vi "saveGraph.vi"(0 "reference":refnum<class "Graph.lvclass">, 1 "filePath":path, 2 "diagramType":T2, 5 "error in (no error)":errorcluster, 6 "ExportType(Normal)":T1) -> (14 "reference out":refnum<class "Graph.lvclass">, 15 "succeeded":bool, 19 "error out":errorcluster)   [LabVIEW 2014, in "Graph.lvclass"]
doc: "Save to File"
uses:
  <resource>/Framework/Providers/Open_GDS/UML/Graph_class/Graph.lvclass
  <resource>/Framework/Providers/Open_GDS/UML/Graph_class/private/diagramType.ctl
  <resource>/Framework/Providers/Open_GDS/UML/Graph_class/SaveTypes.ctl
  <resource>/Framework/Providers/Open_GDS/UML/Graph_class/private/FileSaveVersionType.ctl
  <resource>/Framework/Providers/Open_GDS/UML/AbstractNode_class/AbstractNode.lvclass
  <resource>/Framework/Providers/Open_GDS/UML/AbstractEdge_class/AbstractEdge.lvclass
panel:
  in  "Old":bool
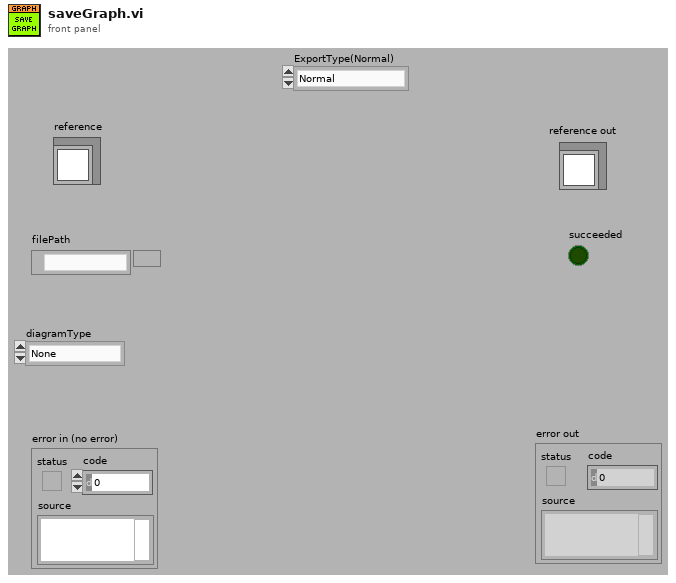
[diagram p1: front panel]
types:
  T1 = typedef "Graph.lvclass/SaveTypes.ctl" = enum16{"Normal", "XMI"}
  T2 = typedef "Graph.lvclass/diagramType.ctl" = enum16{"None", "Class", "Sequency", "State", "UseCase", "DQMH-Module"}
  T3 = cluster{"nodeInfo":cluster{"NodeType":string[], "ParentIndex":i32[], "ChildernIndexies":cluster{i32[]}[], "FlattenData":string[]}, "edgeInfo":cluster{"EdgeType":string[], "StartNodeIndex":i32[], "EndNodeIndex":i32[], "FlattenData":string[]}, "Succeeded":bool, "DiagramData":string}
  T4 = typedef "Graph.lvclass/ObjectAttributes.ctl" = cluster{"nodes":refnum<class "AbstractNode.lvclass">[], "edges":refnum<class "AbstractEdge.lvclass">[], "nodesToBeRemoved":refnum<class "AbstractNode.lvclass">[], "edgesToBeRemoved":refnum<class "AbstractEdge.lvclass">[], "needsLayout":bool, "LayoutNodes":refnum<class "AbstractNode.lvclass">[]}
  T5 = cluster{"children":refnum<class "AbstractNode.lvclass">[]}
  T6 = cluster{"NodeType":string[], "ParentIndex":i32[], "ChildernIndexies":cluster{i32[]}[], "FlattenData":string[]}
  T7 = cluster{"EdgeType":string[], "StartNodeIndex":i32[], "EndNodeIndex":i32[], "FlattenData":string[]}
  T8 = typedef "Graph.lvclass/FileSaveVersionType.ctl" = enum16{"A", "B"}
  T9 = cluster{"TYPEDEF-FileSaveVersion":T8, "diagramType":T2, "DiagramData":string, "nodeInfo":cluster{"NodeType":string[], "ParentIndex":i32[], "ChildernIndexies":cluster{i32[]}[], "FlattenData":string[]}, "edgeInfo":cluster{"EdgeType":string[], "StartNodeIndex":i32[], "EndNodeIndex":i32[], "FlattenData":string[]}}
  T10 = cluster{"diagramType":T2, "nodeInfo":cluster{"NodeType":string[], "ParentIndex":i32[], "ChildernIndexies":cluster{i32[]}[], "FlattenData":string[]}, "edgeInfo":cluster{"EdgeType":string[], "StartNodeIndex":i32[], "EndNodeIndex":i32[], "FlattenData":string[]}}
  T11 = enum16{"open", "replace", "create", "open or create", "replace or create", "replace or create with confirmation"}
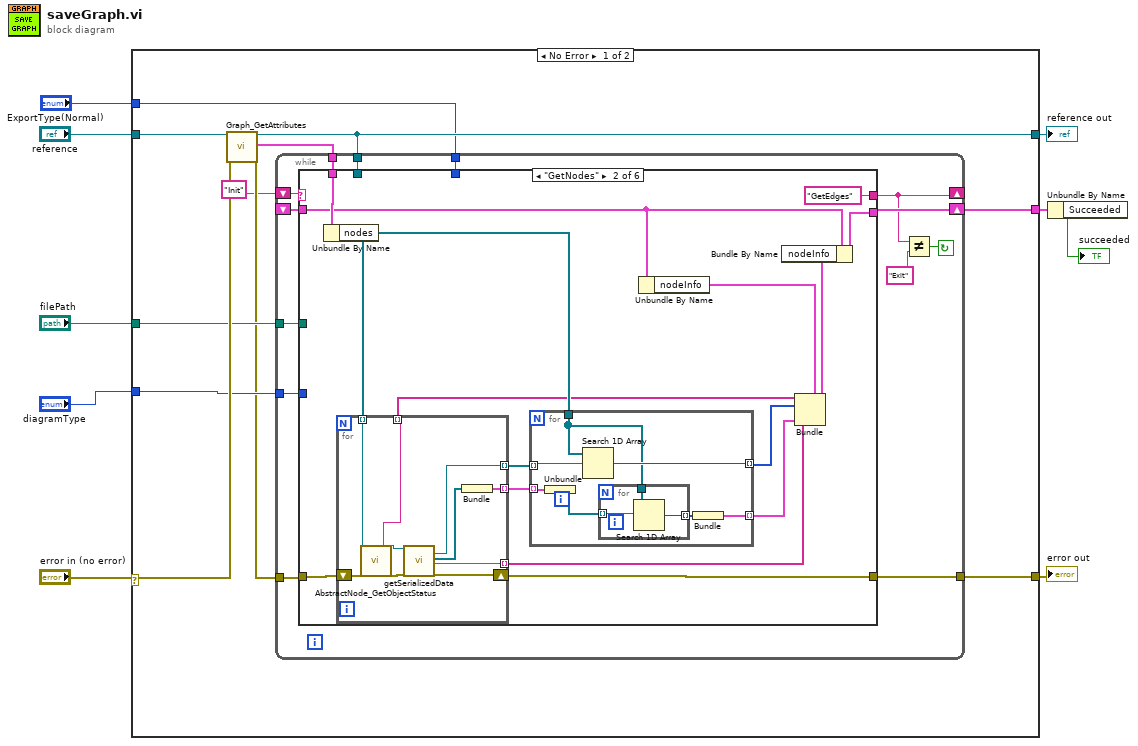
[diagram p0: block diagram]
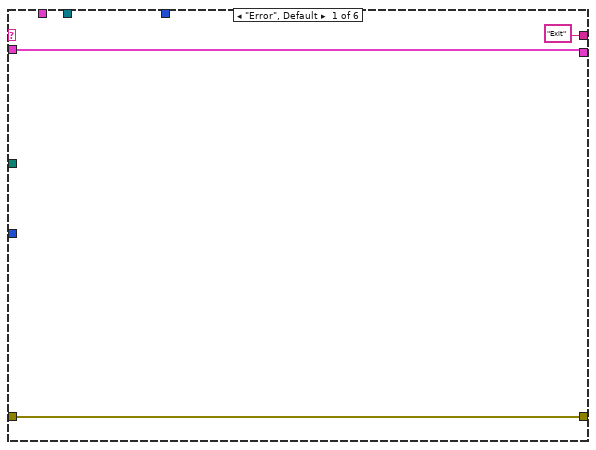
[diagram p2: hidden frame]
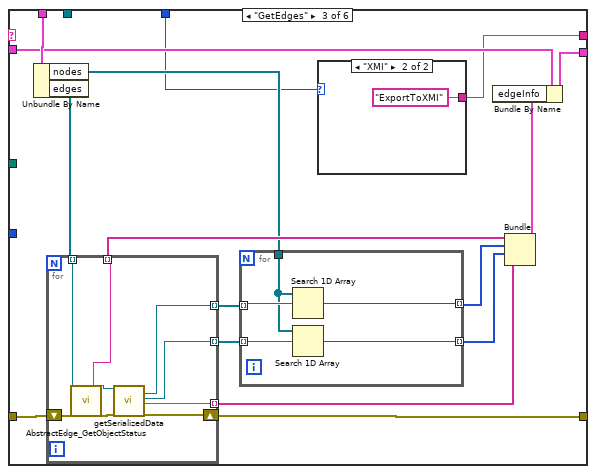
[diagram p3: hidden frame]
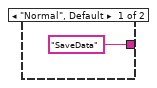
[diagram p4: hidden frame]
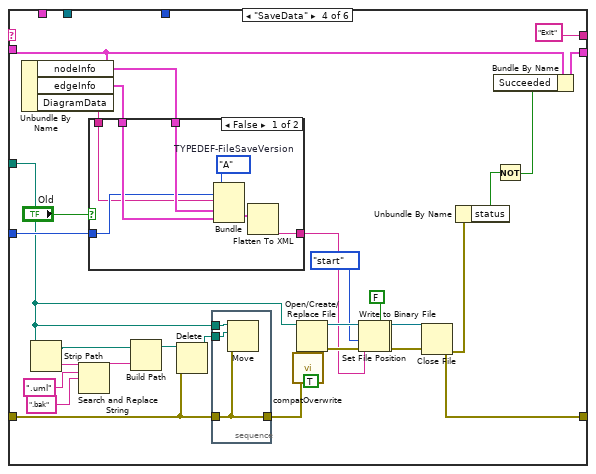
[diagram p5: hidden frame]
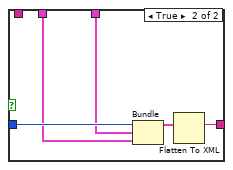
[diagram p6: hidden frame]
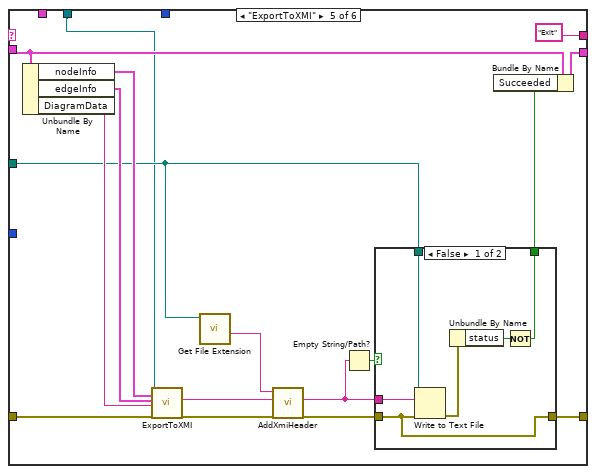
[diagram p7: hidden frame]
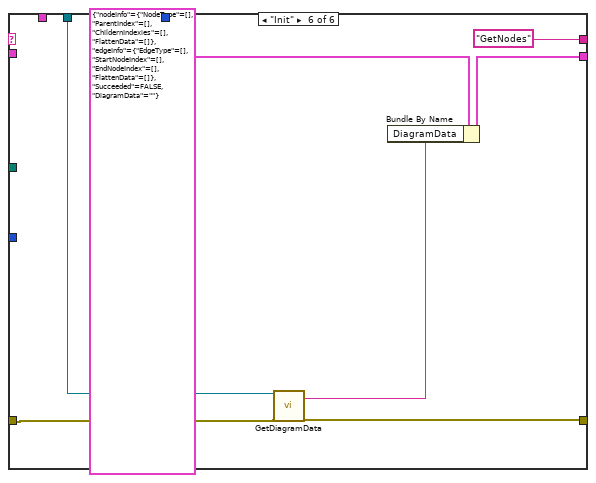
[diagram p9: hidden frame]
diagram:
  n1 = case shown="No Error" "error in (no error)" {
    selector: "error in (no error)" -> [w17 w180]
    tunnel: "reference" -> [w20 w181]
    tunnel: [w19 w180] -> w8
    tunnel: [w18 w181] -> w7
    tunnel: "filePath" -> [w16 _]
    tunnel: "diagramType" -> [w15 _]
    tunnel: [w14 _] -> w3
    tunnel: "ExportType(Normal)" -> [w13 _]
    frame No Error {
      n2 = call <resource>:"Graph_GetAttributes.vi"("reference in"=w20, "error in (no error)"=w17) -> ("reference out"=w18:refnum<class "Graph.lvclass">, "Data"=w10:T4, "error out"=w12:errorcluster)  [unwired: 1 in, 14 out]
      n3 = while {
        tunnel: w10 -> [w33]
        tunnel: w12 -> [w32]
        tunnel: w15 -> [w31]
        tunnel: w16 -> [w30]
        tunnel: [w29] -> w19
        shift-right: [w24] -> _
        shift-left: "Init" -> [w28]
        shift-right: [w27] -> w14
        shift-left: _ -> [w23]
        tunnel: w18 -> [w22]
        tunnel: w13 -> [w21]
        stop <- w25 continue-if-true
        n4 = case shown="\"GetNodes\"" w28 {
          tunnel: w33 -> [_ w51 w86 _ _ _]
          tunnel: w32 -> [w36 w50 w85 w111 w162 w176]
          tunnel: w31 -> [_ _ _ w132 _ _]
          tunnel: w30 -> [_ _ _ w109 w151 _]
          tunnel: [w36 w44 w81 w125 w157 w175] -> w29
          tunnel: [w34 w40 w77 w121 w164 w177] -> w27
          tunnel: ["Exit" ("y") "GetEdges" w71 "Exit" ("y") "Exit" ("y") "GetNodes"] -> w24
          tunnel: w23 -> [w34 w38 w79 w120 w163 _]
          tunnel: w22 -> [_ _ _ _ w149 w173]
          tunnel: w21 -> [_ _ w72 _ _ _]
          frame "Error", Default {
          }
          frame "GetNodes" {
            n5 = Unbundle By Name(w51) -> ("nodes"=w43:refnum<class "AbstractNode.lvclass">[])
            n6 = for {
              shift-right: [w63] -> w44
              shift-left: w50 -> [w70]
              tunnel: w43 -> [w66] mode=indexing
              tunnel: [w69] -> w49 mode=indexing
              tunnel: [w67] -> w48 mode=indexing
              tunnel: [w64] -> w45 mode=indexing
              tunnel: [w62] -> w42 mode=indexing
              n7 = call <resource>:"AbstractNode_GetObjectStatus.vi"("reference in"=w66) -> ("Class name"=w62:string, "reference out"=w65:refnum<class "AbstractNode.lvclass">)  [unwired: 1 in, 16 out]
              n8 = call-dynamic "getSerializedData.vi"("reference"=w65, "error in (no error)"=w70) -> ("parent"=w69:refnum<class "AbstractNode.lvclass">, "children"=w68:refnum<class "AbstractNode.lvclass">[], "xmlOut"=w64:string, "error out"=w63:errorcluster)  [unwired: 13 in, 1 out]
              n9 = Bundle("children"=w68) -> (w67:T5)  [unwired: 1 in]
            }
            n10 = for {
              tunnel: w49 -> [w57] mode=indexing
              tunnel: w48 -> [w58] mode=indexing
              tunnel: [w56] -> w47 mode=indexing
              tunnel: [w53] -> w46 mode=indexing
              tunnel: w43 -> [w52]
              n11 = Unbundle(w58) -> ("children"=w55:refnum<class "AbstractNode.lvclass">[])
              n12 = Search 1D Array(1D array=w52, element=w57) -> (index of element=w56:i32)  [unwired: 1 out]
              n13 = for {
                tunnel: w55 -> [w60] mode=indexing
                tunnel: w52 -> [w61]
                tunnel: [w59] -> w54 mode=indexing
                n14 = Search 1D Array(1D array=w61, element=w60) -> (index of element=w59:i32)  [unwired: 1 out]
              }
              n15 = Bundle(w54) -> (w53:cluster{i32[]})  [unwired: 1 in]
            }
            n16 = Unbundle By Name(w38) -> ("nodeInfo"=w37:T6)
            n17 = Bundle(cluster=w37, "NodeType"=w42, "ParentIndex"=w47, "ChildernIndexies"=w46, "FlattenData"=w45) -> (w41:T6)
            n18 = Bundle By Name(cluster=w38, "nodeInfo"=w41) -> (w40:T3)
          }
          frame "GetEdges" {
            n19 = Unbundle By Name(w86) -> ("nodes"=w76:refnum<class "AbstractNode.lvclass">[], "edges"=w75:refnum<class "AbstractEdge.lvclass">[])
            n20 = for {
              shift-right: [w95] -> w81
              shift-left: w85 -> [w101]
              tunnel: w75 -> [w99] mode=indexing
              tunnel: [w100] -> w84 mode=indexing
              tunnel: [w96] -> w82 mode=indexing
              tunnel: [w94] -> w80 mode=indexing
              tunnel: [w97] -> w74 mode=indexing
              n21 = call <resource>:"AbstractEdge_GetObjectStatus.vi"("reference in"=w99) -> ("Class name"=w94:string, "reference out"=w98:refnum<class "AbstractEdge.lvclass">)  [unwired: 1 in, 16 out]
              n22 = call-dynamic "getSerializedData.vi"("reference"=w98, "error in (no error)"=w101) -> ("startNode"=w100:refnum<class "AbstractNode.lvclass">, "endNode"=w97:refnum<class "AbstractNode.lvclass">, "xmlOut"=w96:string, "error out"=w95:errorcluster)  [unwired: 13 in, 1 out]
            }
            n23 = for {
              tunnel: w84 -> [w93] mode=indexing
              tunnel: [w92] -> w83 mode=indexing
              tunnel: w76 -> [w91]
              tunnel: w74 -> [w90] mode=indexing
              tunnel: [w89] -> w73 mode=indexing
              n24 = Search 1D Array(1D array=w91, element=w93) -> (index of element=w92:i32)  [unwired: 1 out]
              n25 = Search 1D Array(1D array=w91, element=w90) -> (index of element=w89:i32)  [unwired: 1 out]
            }
            n26 = case shown="\"XMI\"" w72 {
              tunnel: ["SaveData" "ExportToXMI"] -> w71
              frame "Normal", Default {
              }
              frame "XMI" {
              }
            }
            n27 = Bundle(w80, w83, w73, w82) -> (w78:cluster{string[], i32[], i32[], string[]})  [unwired: 1 out]
            n28 = Bundle By Name(cluster=w79, "edgeInfo"=w78) -> (w77:T3)
          }
          frame "SaveData" {
            n29 = Unbundle By Name(w120) -> ("nodeInfo"=w131:T6, "edgeInfo"=w130:T7, "DiagramData"=w107:string)
            n30 = Strip Path(path=w109) -> (stripped path=w118:path, name=w117:string)
            n31 = Search and Replace String(input string=w117, search string=".uml", replace string=".bak" ("replace string (\"\")")) -> (result string=w114:string)  [unwired: 1 in, 7 out]
            n32 = case shown="False" "Old" {
              tunnel: w132 -> [w137 w145]
              tunnel: w131 -> [w139 w144]
              tunnel: w130 -> [w138 w143]
              tunnel: w107 -> [w134 _]
              tunnel: [w135 w141] -> w106
              frame False {
                w140 = FileSaveVersionType."A"  # TYPEDEF-FileSaveVersion
                n33 = Bundle("TYPEDEF-FileSaveVersion"=w140, "diagramType"=w137, "DiagramData"=w134, "nodeInfo"=w139, "edgeInfo"=w138) -> (w136:T9)  [unwired: 1 out]
                n34 = Flatten To XML(anything=w136) -> (xml string=w135:string)
              }
              frame True {
                n35 = Bundle("diagramType"=w145, "nodeInfo"=w144, "edgeInfo"=w143) -> (w142:T10)  [unwired: 1 out]
                n36 = Flatten To XML(anything=w142) -> (xml string=w141:string)
              }
            }
            n37 = Build Path(base path=w118, name or relative path=w114) -> (appended path=w113:path)
            n38 = Delete(path (use dialog)=w113, error in=w111) -> (deleted path=w112:path)  [unwired: 5 out]
            n39 = stacked-sequence {
              tunnel: w109 -> [w148]
              tunnel: w112 -> [w147]
              tunnel: w111 -> [w146]
              tunnel: [w146] -> w110
              frame #0 {
                n40 = Move(source path=w148, error in=w146, 10:w147) -> ()  [unwired: 5 out]
              }
            }
            n41 = call <vilib>:"compatOverwrite.vi"("overwrite (F)"=TRUE) -> ("overwrite?"=w105:T11)
            n42 = Open/Create/Replace File(file path (use dialog)=w109, error in=w110, operation (0:open)=w105) -> (refnum out=w128:refnum<file>, error out=w129:errorcluster)  [unwired: 3 in, 1 out]
            n43 = Set File Position(refnum=w128, from (0:start)=enum16{"start", "end", "current"}."start" ("pos mode (0:2)"), error in=w129) -> (refnum out=w104:refnum<file>, error out=w103:errorcluster)  [unwired: 1 out]
            n44 = Write to Binary File(file (use dialog)=w104, data=w106, error in=w103, 5:FALSE ("prepend array or string size? (T)")) -> (refnum out=w126:refnum<file>, error out=w127:errorcluster)  [unwired: 3 out]
            n45 = Close File(refnum=w126, error in=w127) -> (error out=w125:errorcluster)  [unwired: 1 out]
            n46 = Unbundle By Name(w125) -> ("status"=w122:bool)
            n47 = Not(x=w122) -> (.not. x?=w119:bool)
            n48 = Bundle By Name(cluster=w120, "Succeeded"=w119) -> (w121:T3)
          }
          frame "ExportToXMI" {
            n49 = Unbundle By Name(w163) -> ("nodeInfo"=w161:T6, "edgeInfo"=w160:T7, "DiagramData"=w159:string)
            n50 = call-dynamic "ExportToXMI.vi"("reference"=w149, "nodeInfo"=w161, "edgeInfo"=w160, "DiagramData"=w159, "error in (no error)"=w162) -> ("XMIText"=w155:string, "error out"=w154:errorcluster)  [unwired: 12 in, 1 out]
            n51 = call <vilib>:"Get File Extension.vi"("file"=w151) -> ("filename without extension"=w150:string)  [unwired: 1 in, 9 out]
            n52 = call <resource>:"AddXmiHeader.vi"("error in (no error)"=w154, "XmiContent"=w155, "DiagramName"=w150) -> ("error out"=w153:errorcluster, "XmiDocument"=w152:string)  [unwired: 7 out]
            n53 = Empty String/Path?(string/path=w152) -> (empty?=w158:bool)
            n54 = case shown="False" w158 {
              tunnel: w153 -> [w169 w172]
              tunnel: [w169 w172] -> w157
              tunnel: [w166 _] -> w156
              tunnel: w151 -> [w171 _]
              tunnel: w152 -> [w170 _]
              frame False {
                n55 = Write to Text File(file (use dialog)=w171, text=w170, error in=w169) -> (error out=w168:errorcluster)  [unwired: 3 out]
                n56 = Unbundle By Name(w168) -> ("status"=w167:bool)
                n57 = Not(x=w167) -> (.not. x?=w166:bool)
              }
              frame True {
              }
            }
            n58 = Bundle By Name(cluster=w163, "Succeeded"=w156) -> (w164:T3)
          }
          frame "Init" {
            n59 = call-dynamic "GetDiagramData.vi"("reference"=w173, "error in (no error)"=w176) -> ("DiagramData"=w174:string, "error out"=w175:errorcluster)  [unwired: 15 in, 1 out]
            n60 = Bundle By Name(cluster=T3 {"nodeInfo"={"NodeType"=[], "ParentIndex"=[], "ChildernIndexies"=[], "FlattenData"=[]}, "edgeInfo"={"EdgeType"=[], "StartNodeIndex"=[], "EndNodeIndex"=[], "FlattenData"=[]}, "Succeeded"=FALSE, "DiagramData"=""}, "DiagramData"=w174) -> (w177:T3)
          }
        }
        n61 = Not Equal?(x=w24, y="Exit") -> (x != y?=w25:bool)
      }
    }
    frame Error {
    }
  }
  "reference out" <- w7
  "error out" <- w8
  n62 = Unbundle By Name(w3) -> ("Succeeded"=→"succeeded":bool)
